vi "GUI_HTT_CTRLv2.vi"() -> ()   [LabVIEW 2013]
uses:
  Shared/GUI_Template/GUI_master/tcp_new_data_event.ctl
  Shared/GUI_Template/GUI_master/tcp new data cluster.ctl
  GUI_TestStand/Fire button.ctl
  <vilib>/Platform/browser.llb/Open URL in Default Browser (string).vi
panel:
  in  "Position.Axis 3::4":dbl caption="Turning M" min=0.0 max=26.0
  in  "Position.Axis 2::4":dbl caption="Delay" min=-20.0 max=48.0
  in  "FilterWheelB1":bool caption="PicoB GUI"
  in  "Search Log":bool caption="PicoL GUI"
  in  "Experiment \n(if, shadow, topjet)":bool caption="PicoL GUI"
  in  "Switcher":bool
  in  "RemoteDesktop":bool caption="PicoL GUI"
  in  "ai_mean.channel 1::13":dbl caption="GenTec" min=0.0 max=0.0 format="%#_6e"
  in  "ai_mean.channel 0::13":dbl caption="Pelliclemeter" min=0.0 max=0.0 format="%#_6e"
  in  "GUIdevice 13":string="HTT_DG645"
  in  "Experiment \n(e-profile, xrays)":bool caption="PicoL GUI"
  in  "IR TC Pointing (17s)":bool caption="PicoL GUI"
  in  "Scatter Depletion":bool caption="PicoL GUI"
  in  "Scatter IR Amps":bool caption="PicoL GUI"
  in  "Drive TC Pt":bool caption="PicoL GUI"
  in  "Gaia Profiles":bool caption="PicoL GUI"
  in  "Gaia Pointing":bool caption="PicoL GUI"
  in  "IR Exp and Comp":bool caption="PicoL GUI"
  in  "HTT Interactive":bool caption="PicoL GUI"
  in  "GUIdevice 12":string="HTT_DG645"
  in  "Delay.Ch C::12":dbl caption="Delay" min=-0.1 max=2.0 format="%#_6e"
  in  "Delay.Ch D::12":dbl caption="Width" min=-0.1 max=2.0 format="%#_6e"
  in  "Amplitude.Ch CD::12":dbl caption="DG645" min=0.5 max=5.0
  in  "Field::1":dbl caption="B-Field" min=0.0 max=10000.0
  in  "Delay.Ch 1::8":dbl caption="Delay" min=0.0 max=10.0 format="%#_6e"
  in  "Width.Ch 1::8":dbl caption="Width" min=0.0 max=1.0 format="%#_6e"
  in  "Amplitude.Ch 1::8":dbl caption="Cam Trig Amp" min=0.0 max=12.0
  in  "Position.Axis 2::6":dbl caption="Prepulse delay" min=-6000.0 max=6000.0
  in  "1Wire GUI":bool caption="PicoL GUI"
  in  "Opt. Spectrometer":bool caption="PicoL GUI"
  in  "SingleCamGUI":bool caption="PicoL GUI"
  in  "Exp Editor":bool caption="PicoL GUI"
  in  "DB Editor":bool caption="PicoL GUI"
  in  "AddColumns":bool caption="PicoL GUI"
  in  "GEECSplot":bool caption="PicoL GUI"
  in  "LVStarter":bool caption="PicoL GUI"
  in  "MasterControl":bool caption="PicoL GUI"
  in  "MagSpecGUI":bool caption="PicoL GUI"
  in  "DailyLog":bool caption="PicoL GUI"
  in  "EnTempLogger":bool caption="PicoL GUI"
  in  "Depletion Cams":bool caption="PicoL GUI"
  in  "D-L-Cams":bool caption="PicoL GUI"
  in  "Position.Axis 2::5":dbl caption="Mode Out z" min=-150.0 max=150.0
  in  "Position.Axis 1::4":dbl caption="Blade" min=-20.0 max=20.0
  out "Temperature::11":dbl caption="Temp Amps" min=0.0 max=500.0 format="%#_3f"
  out "Temperature::10":dbl caption="Temp Gaia" min=0.0 max=500.0 format="%#_3f"
  out "Energy.Channel 0::7":dbl caption="IR Splitmeter" min=0.0 max=20.0 format="%#_3e"
  in  "Amplitude.Ch 5::8":dbl caption="Trigger Amplitude" min=0.0 max=12.0
  in  "Position.Axis 3::5":dbl caption="Mode In z" min=-200.0 max=200.0
  in  "Position.Axis 1::5":dbl caption="Mode Out Wedge" min=-150.0 max=150.0
  out "Position.Axis3::2":dbl caption="Rotation G1" min=-180.0 max=180.0 format="%#_13g"
  out "Position.Axis2::2":dbl caption="Rotation G2" min=-180.0 max=180.0 format="%#_13g"
  in  "Position.Axis1::2":dbl caption="Translation" min=-60000.0 max=60000.0 format="%#_13g"
  in  "PicoL":bool caption="PicoL GUI"
  in  "PicoB":bool caption="PicoB GUI"
  in  "AnalogOutput.Channel 0::9":dbl caption="Pressure Ctrl (V)" min=0.0 max=10.0
  in  "Width.Ch 5::8":dbl caption="Opening time (s)" min=0.0 max=0.025 format="%#_6e"
  in  "Jet enable":bool caption="Jet Enable"
  in  "Jet trigger":bool caption="Jet Trigger"
  in  "Position.Axis 3::3":dbl caption="Jet Z" min=-25.0 max=25.0
  in  "Position.Axis 2::3":dbl caption="Jet Y" min=-25.0 max=25.0
  in  "Position.Axis 1::3":dbl caption="Jet X" min=-25.0 max=25.0
  in  "Position.Axis 3::6":dbl caption="Probe delay" min=-76.0 max=76.0
  in  "GUIdevice 11":string="HTT-Temp-Amps"
  in  "GUIdevice 8":string="HTT-BNC"
  in  "GUIdevice 6":string="HTT-ESP04"
  in  "GUIdevice 5":string="HTT-ESP03"
  in  "Fire Button":T1=TRUE
  out "error IO 2":errorcluster
  out "fire::10":string
  out "tcp data event":T2
  in  "UDP error message":string
  in  "GUIdevice 7":string="HTT-Pulsar"
  in  "GUIdevice 2":string="Aerotech-HTT"
  in  "GUIdevice 10":string="HTT-Temp-Gaia"
  in  "GUIdevice 4":string="HTT-ESP02"
  in  "GUIdevice 1":string="HTT-MagTeslameter-DTM141"
  in  "GUIdevice 3":string="HTT-ESP01"
  in  "GUIdevice 9":string="HTT-HighPressureDAQ"
  in  "Delay.Ch 5::8":dbl caption="Jet timing (s)" min=0.0 max=10.0 format="%#_6e"
  in  "stop":bool
  # "Energy"
  # "CAP"
  # "HTT CONTROL CENTER"
  # "Drive"
  # "Gas Jet"
  # "GUI Collection"
  # "Drive Cameras"
  # "Compressor"
  # "Mode Imager"
  # "Scatter Cameras"
  # "Scatter"
  # "Electronics"
  # "BNC"
  # "Experiment GUIs"
  # "MC Links"
  # "Documentation"
  # "Adjustment GUIs"
  # "Energy Measurements"
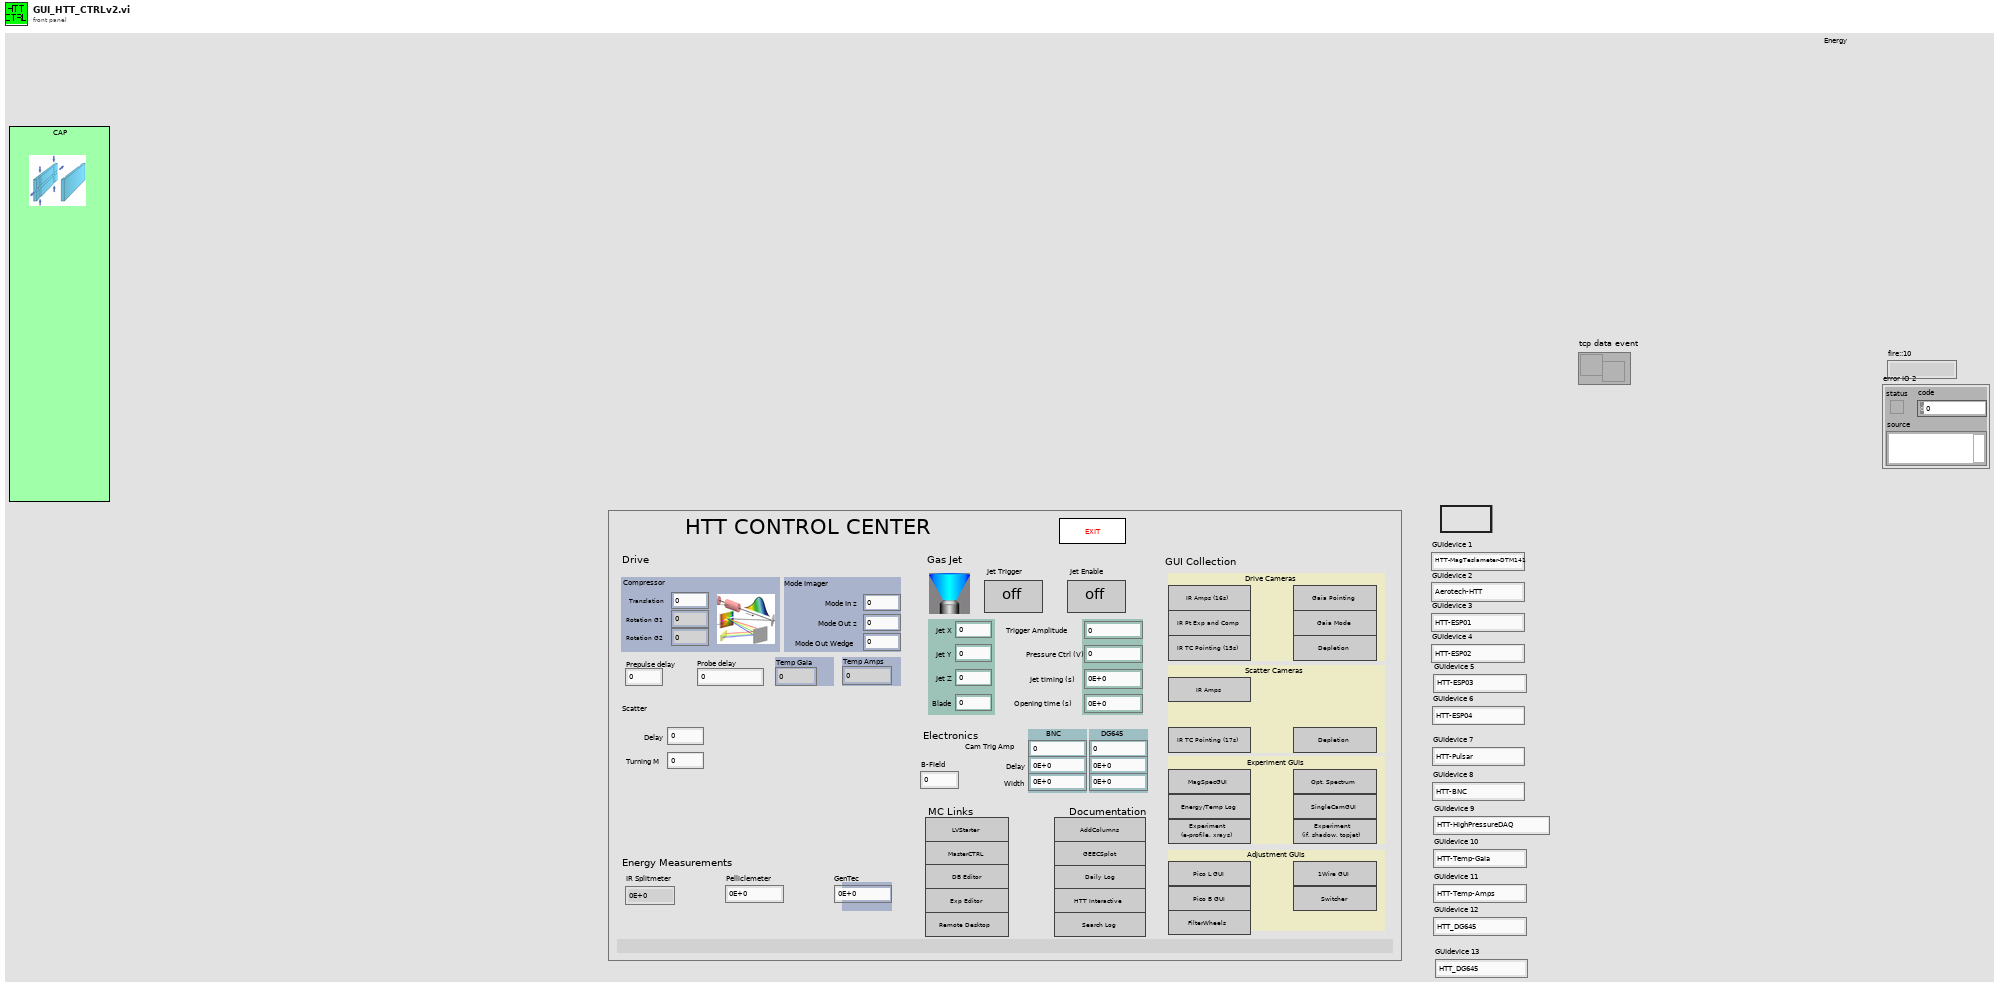
[diagram p1: front panel]
types:
  T1 = typedef "Fire button.ctl" = bool
  T2 = typedef "tcp_new_data_event.ctl" = refnum<user-event>
  T3 = typedef "tcp new data cluster.ctl" = cluster{"EventEnum":enum16{"new data", "connection status update"}, "Device name":string}
  T4 = enum32{"invalid app kind", "Development System", "Run Time System", "Student Edition", "Embedded LabVIEW", "Evaluation", "Custom"}
  T5 = enum32{"Invalid", "Standard", "Closed", "Hidden", "Minimized", "Maximized"}
  T6 = cluster{"Core":cluster{"Current VI Reference":refnum<vi>, "Close Panel on Exit?":bool}, "Heater timing offset":dbl, "Discharge timing offset":dbl, "Jet trigger":bool, "Tik1":u32, "Tik2":u32, "Fire Continues Allowed":bool, "Jet enable":bool}
  T7 = cluster{"Current VI Reference":refnum<vi>, "Close Panel on Exit?":bool}
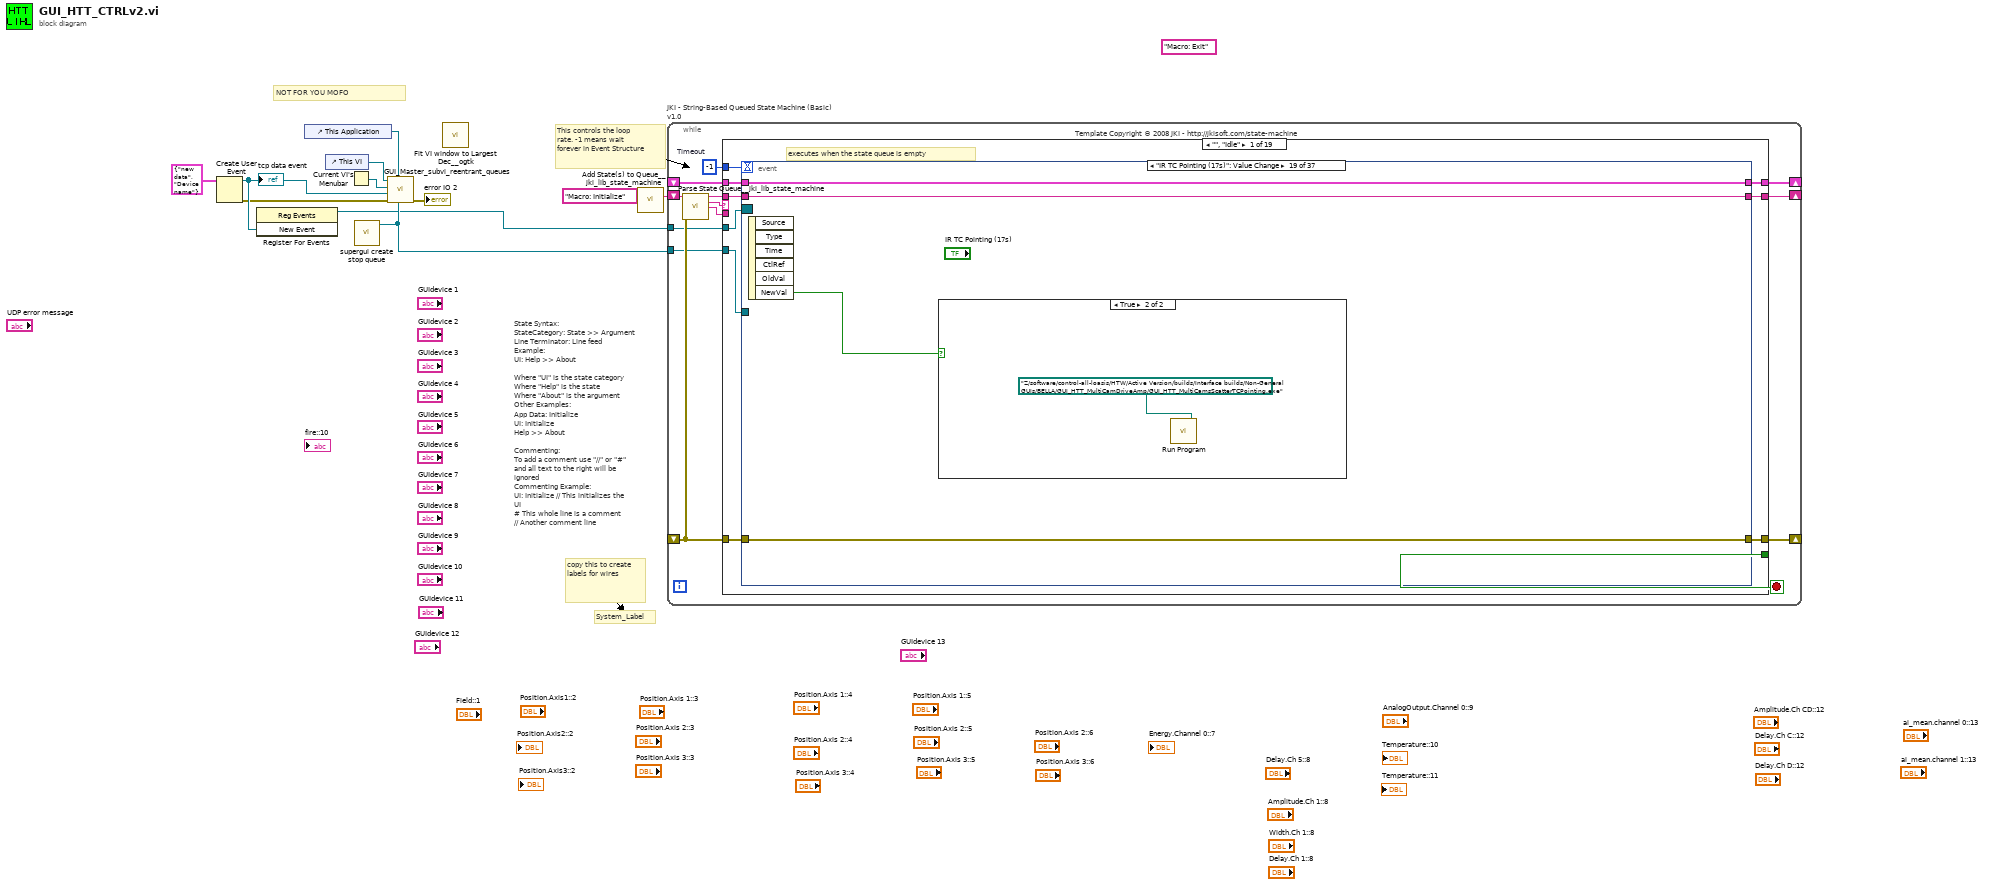
[diagram p0: block diagram]
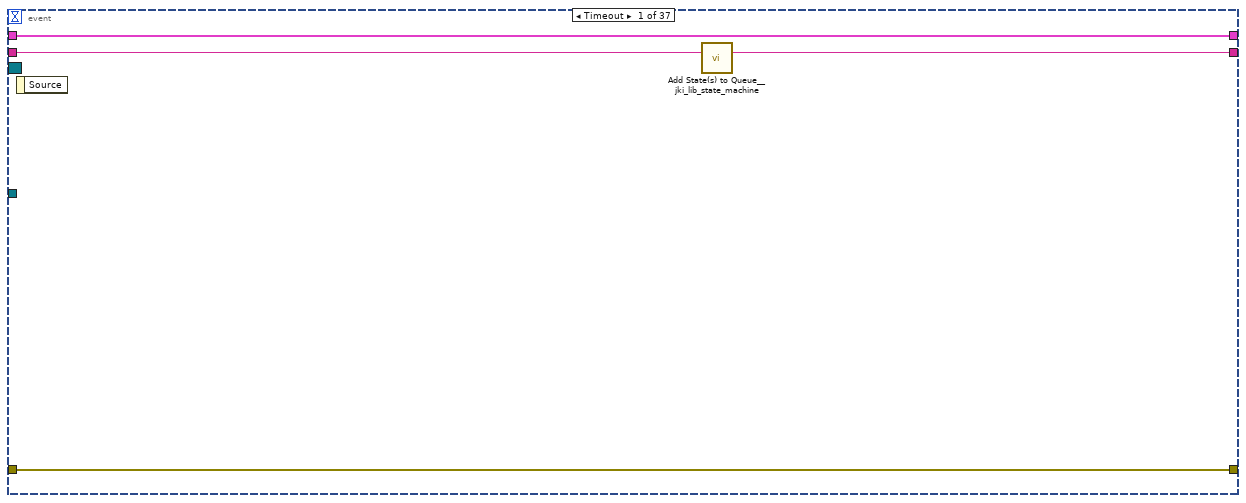
[diagram p2: hidden frame]
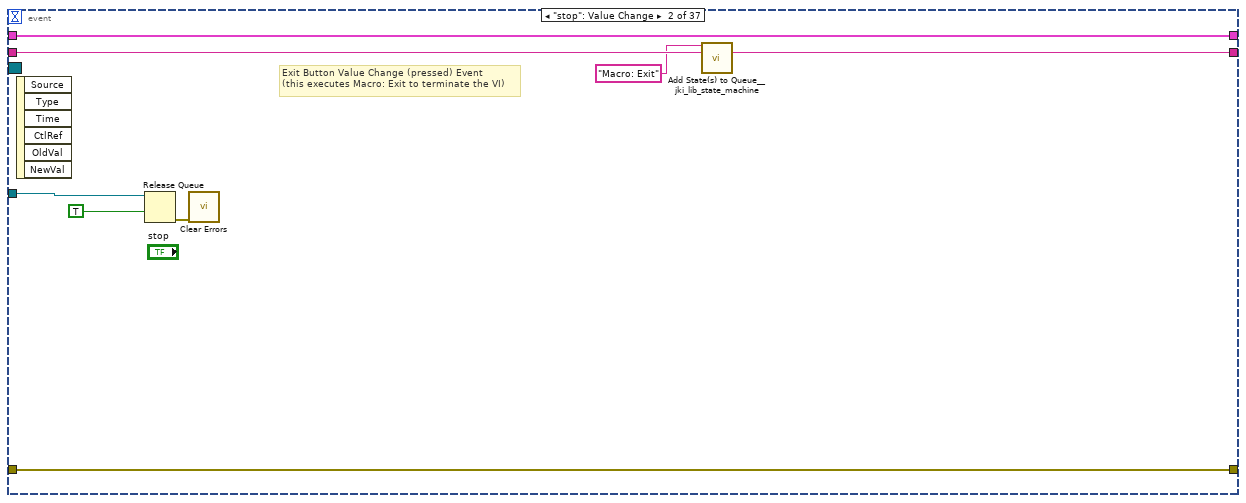
[diagram p3: hidden frame]
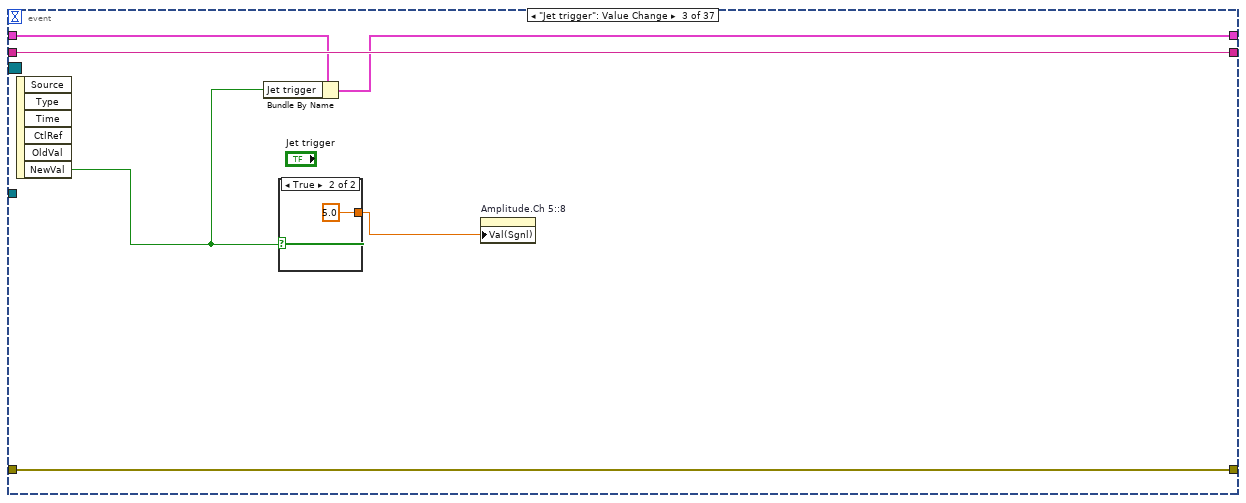
[diagram p4: hidden frame]
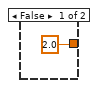
[diagram p5: hidden frame]
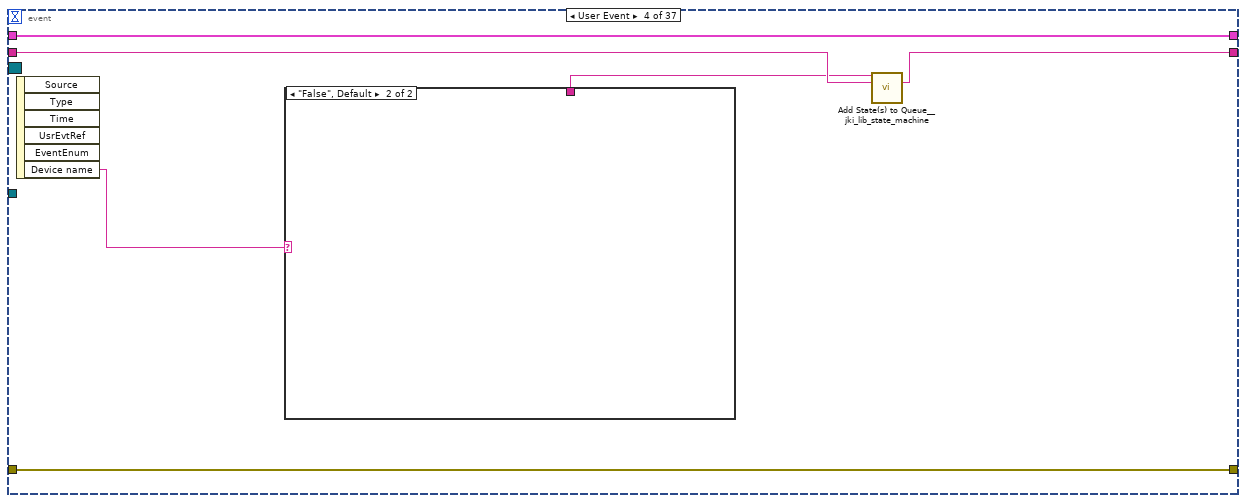
[diagram p6: hidden frame]
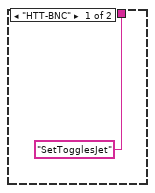
[diagram p7: hidden frame]
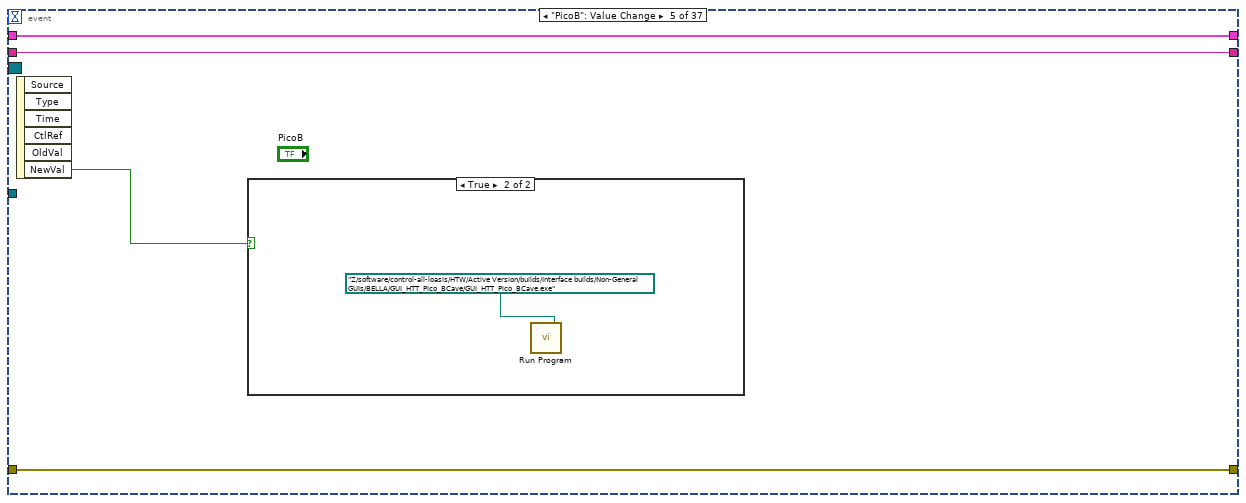
[diagram p8: hidden frame]
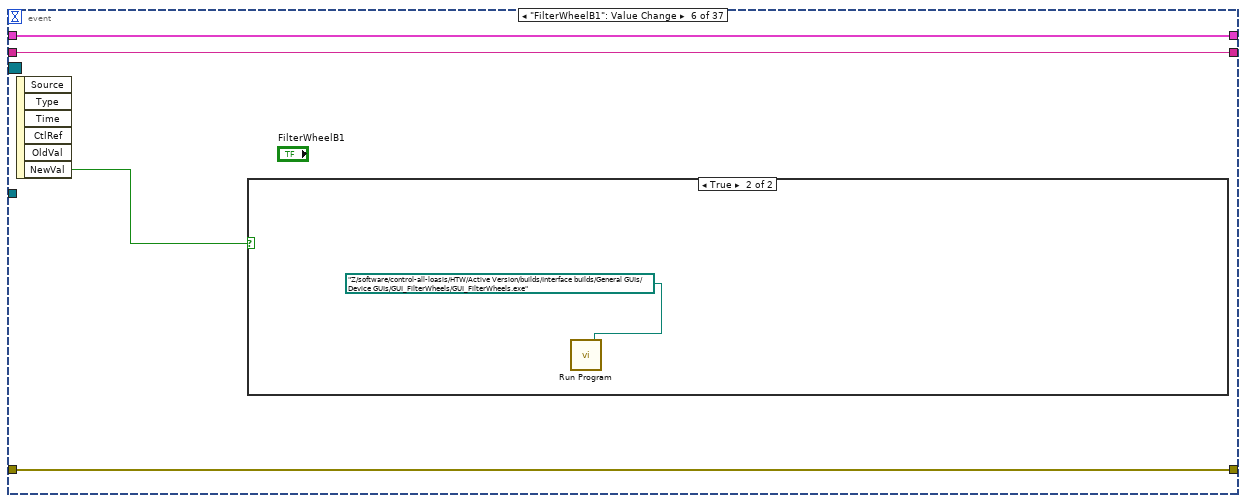
[diagram p10: hidden frame]
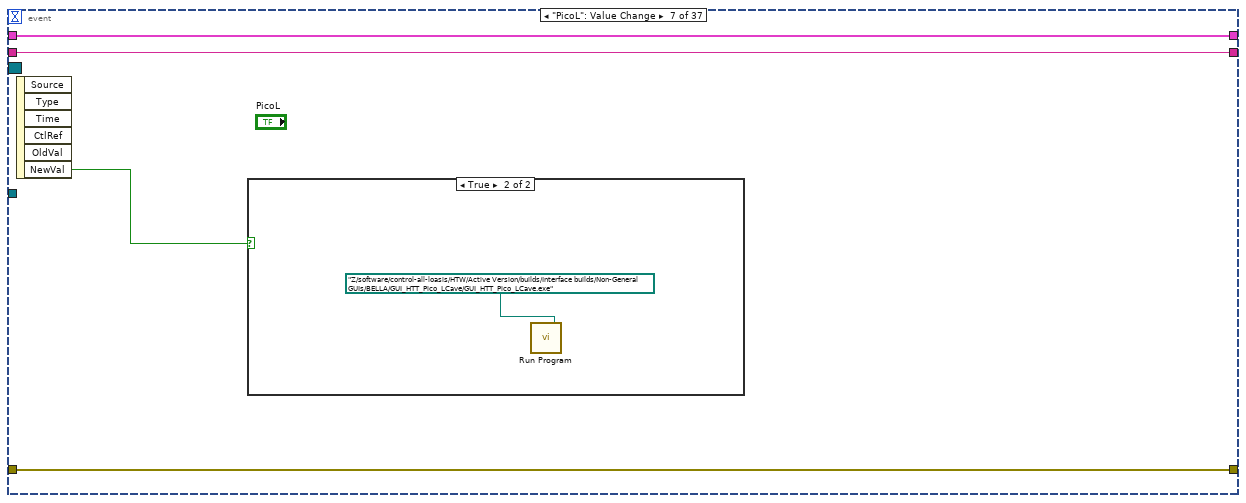
[diagram p12: hidden frame]
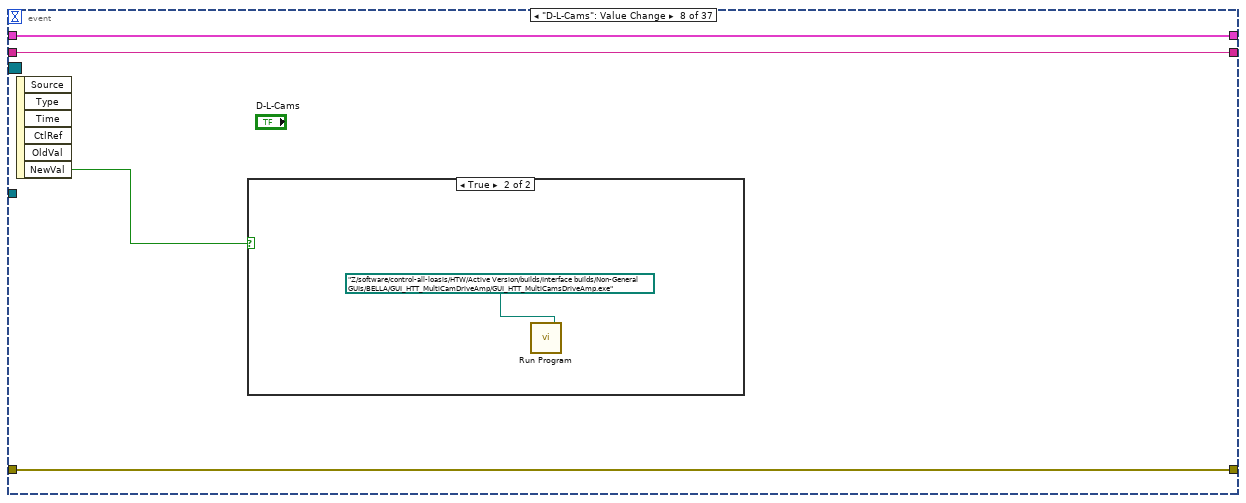
[diagram p14: hidden frame]
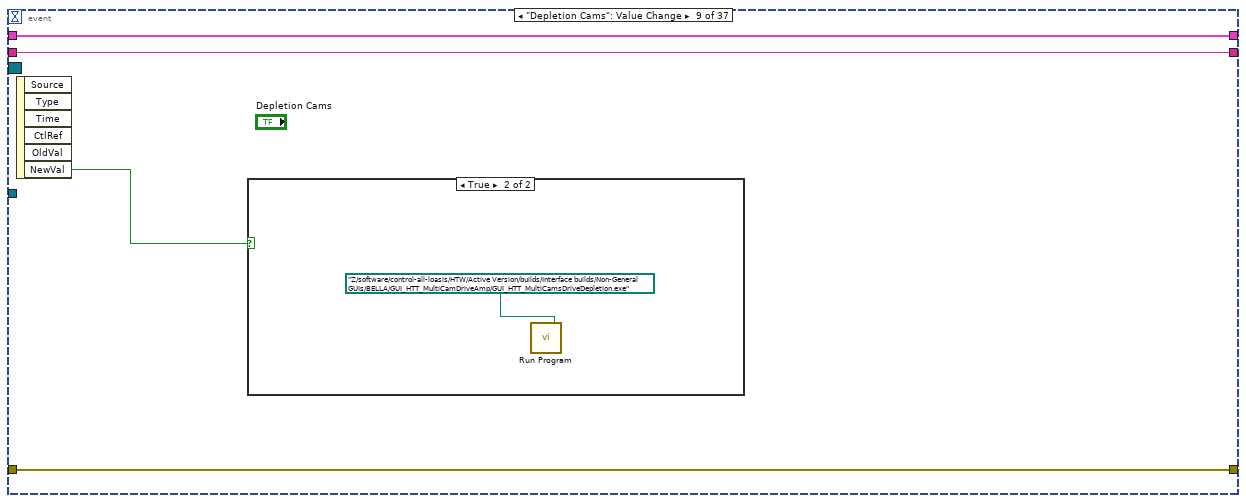
[diagram p16: hidden frame]
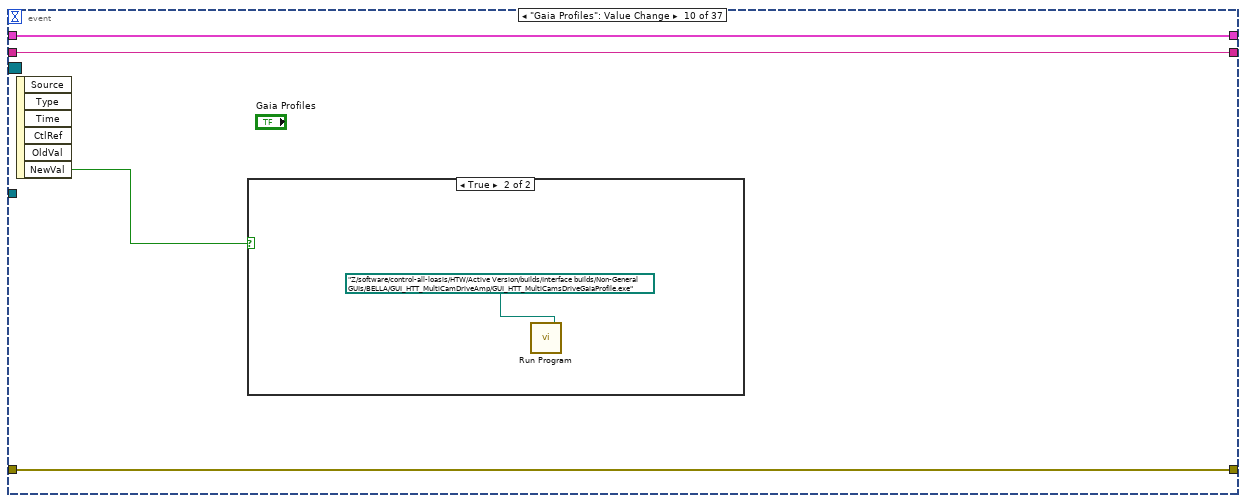
[diagram p18: hidden frame]
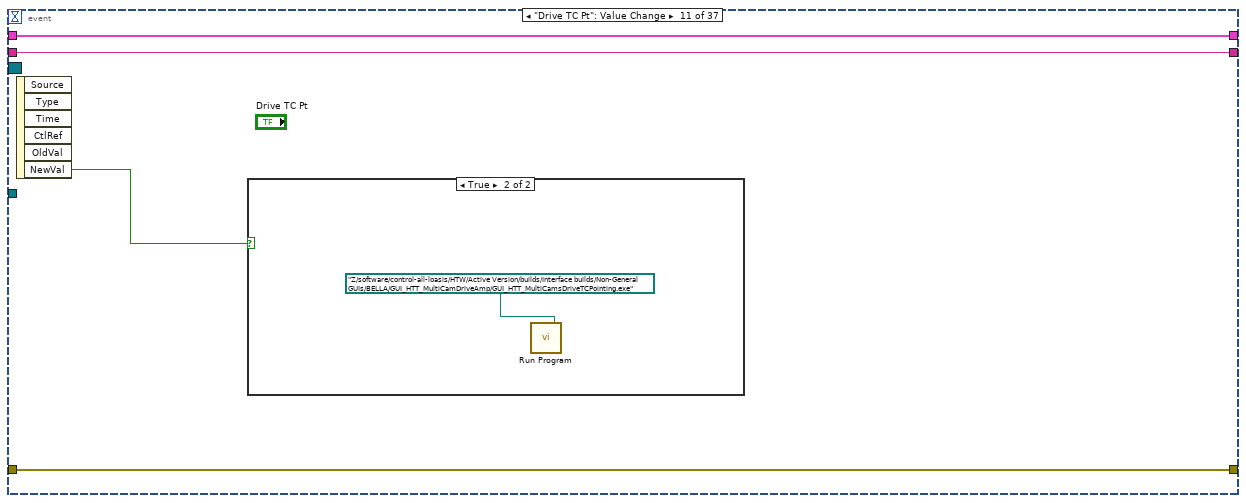
[diagram p20: hidden frame]
diagram:
  (unwired) "Macro: Exit"
  # "State Syntax:\nStateCategory: State >> Argument\nLine Terminator: Line feed\nExample:\nUI: Help >> About\n\nWhere \"UI\" is the state category\nWhere \"Help\" is the state\nWhere \"About\" is the argument\nOther Examples:\nApp Data: Initialize\nUI: Initialize\nHelp >> About\n\nCommenting:\nTo add a comment use \"//\" or \"#\" and all text to the right will be ignored\nCommenting Example:\nUI: Initialize // This initializes the UI\n# This whole line is a comment\n// Another comment line"
  # "copy this to create labels for wires"
  # "This controls the loop rate. -1 means wait forever in Event Structure"
  # "System_Label"
  # "NOT FOR YOU MOFO"
  n1 = Create User Event(user event datatype=T3 {"EventEnum"=enum."new data", "Device name"="Device name"} ("New Event")) -> (user event=w10:refnum<user-event>, error out=w9:errorcluster)  [unwired: 1 in]
  "tcp data event" <- w10
  n2 = register-events(w10) -> (reference out=w1:refnum<event-registration>)  [unwired: 2 in, 1 out]
  n3 = control-ref of="This Application"() -> (w11:refnum<vi>)
  n4 = control-ref of="This VI"() -> (w5:refnum<vi>)
  n5 = Current VI's Menubar() -> (w7:refnum<k9>)
  n6 = call "supergui create stop queue.vi"() -> ("STOP Queue out"=w2:refnum<queue>)  [unwired: 11 in]
  n7 = call "GUI_Master_subvi_reentrant_queues.vi"("STOP Queue in"=w2, "This Application"=w11, "error in (no error)"=w9, "tcp data event"=w10, "Caller menu reference"=w7, "Caller VI ref"=w5) -> ("error out"=→"error IO 2":errorcluster)  [unwired: 5 in]
  n8 = call <userlib>:"Fit VI window to Largest Dec__ogtk.vi"() -> ()  [unwired: 6 in, 2 out]
  n9 = call <vilib>:"Add State(s) to Queue__jki_lib_state_machine.vi"("State(s) in (\"\")"="Macro: Initialize") -> ("States Out"=w3:string)  [unwired: 14 in]
  n10 = while "JKI - String-Based Queued State Machine (Basic) v1.0" {
    shift-right: [w17] -> _
    shift-left: _ -> [w16]
    shift-right: [w20] -> _
    shift-left: _ -> [w14]
    shift-right: [w19] -> _
    shift-left: w3 -> [w21]
    tunnel: w1 -> [w13]
    tunnel: w2 -> [w12]
    stop <- w18 stop-if-true
    w15 = -1  # Timeout
    # "Template Copyright © 2008 JKI - http://jkisoft.com/state-machine"
    n11 = call <vilib>:"Parse State Queue__jki_lib_state_machine.vi"("State Queue"=w21, "Error In (no error)"=w14) -> ("Remaining States"=w23:string, "Current State"=w24:string, "Arguments"=w22:string)  [unwired: 11 in]
    n12 = case shown="\"\", \"Idle\"" w24 {
      selector: w24 -> [_ _ _ w249 _ _ _ _ _ _ _ _ _ _ _ _ _ _ _]
      tunnel: w23 -> [w33 w243 w248 w253 w271 w277 w282 w286 w298 w304 w308 w312 w318 w329 w355 w360 w370 w374 w380]
      tunnel: w22 -> [_ _ _ _ _ _ _ _ _ _ _ _ w313 w323 _ _ _ _ _]
      tunnel: w16 -> [w31 w244 w245 w251 w262 w274 w280 w283 _ w299 w305 w310 w316 w325 w352 w357 w367 w371 w378]
      tunnel: [w30 w242 w246 w255 w268 errorcluster {"status"=FALSE, "code"=0, "source"=""} ("error out") w279 w284 w295 w300 w306 w309 w314 w326 w353 w358 w368 w372 w375] -> w20
      tunnel: w14 -> [w29 w242 w246 w254 w268 w273 w279 w284 w295 w301 w306 w309 w315 w327 w353 w358 w368 w372 w376]
      tunnel: [w32 w243 w247 w252 w270 w276 w281 w285 w297 w303 w307 w311 w317 w328 w354 w359 w369 w373 w379] -> w19
      tunnel: [_ _ _ _ _ _ TRUE _ _ _ _ _ _ _ _ _ _ _ _] -> w18
      tunnel: [w25 w244 w245 w251 w269 w274 w280 w283 w296 w299 w305 w310 w316 w325 w352 w357 w367 w371 w378] -> w17
      tunnel: w15 -> [w28 _ _ _ _ _ _ _ _ _ _ _ _ _ _ _ _ _ _]
      tunnel: w13 -> [w27 _ _ _ _ _ _ _ _ _ _ _ _ _ _ _ _ _ _]
      tunnel: w12 -> [w26 _ _ _ _ _ _ _ _ _ _ _ _ _ _ _ _ _ _]
      frame "", "Idle" {
        # "executes when the state queue is empty"
        n13 = event shown="[18] \"IR TC Pointing (17s)\": Value Change" {
          selector: w27 -> [_ _ _ _ _ _ _ _ _ _ _ _ _ _ _ _ _ _ _ _ _ _ _ _ _ _ _ _ _ _ _ _ _ _ _ _ _]
          dyn-events: _ -> [_ _ _ _ _ _ _ _ _ _ _ _ _ _ _ _ _ _ _ _ _ _ _ _ _ _ _ _ _ _ _ _ _ _ _ _ _]
          timeout: w28 -> [_ _ _ _ _ _ _ _ _ _ _ _ _ _ _ _ _ _ _ _ _ _ _ _ _ _ _ _ _ _ _ _ _ _ _ _ _]
          tunnel: w33 -> [w37 w45 w51 w57 w64 w69 w74 w79 w84 w89 w94 w99 w104 w109 w114 w119 w124 w129 w134 w139 w144 w149 w154 w159 w164 w169 w174 w179 w184 w189 w194 w199 w204 w209 w216 w220 w229]
          tunnel: [w36 w44 w51 w56 w64 w69 w74 w79 w84 w89 w94 w99 w104 w109 w114 w119 w124 w129 w134 w139 w144 w149 w154 w159 w164 w169 w174 w179 w184 w189 w194 w199 w204 w209 w216 w221 w228] -> w32
          tunnel: w31 -> [w34 w42 w50 w58 w61 w66 w71 w76 w81 w86 w91 w96 w101 w106 w111 w116 w121 w126 w131 w136 w141 w146 w151 w156 w161 w166 w171 w176 w181 w186 w191 w196 w201 w206 w215 w223 w226]
          tunnel: [w35 w43 w47 w55 w62 w67 w72 w77 w82 w87 w92 w97 w102 w107 w112 w117 w122 w127 w132 w137 w142 w147 w152 w157 w162 w167 w172 w177 w182 w187 w192 w197 w202 w207 w211 w222 w227] -> w30
          tunnel: w29 -> [w35 w43 w47 w55 w62 w67 w72 w77 w82 w87 w92 w97 w102 w107 w112 w117 w122 w127 w132 w137 w142 w147 w152 w157 w162 w167 w172 w177 w182 w187 w192 w197 w202 w207 w211 w222 w227]
          tunnel: [w34 w42 w49 w58 w61 w66 w71 w76 w81 w86 w91 w96 w101 w106 w111 w116 w121 w126 w131 w136 w141 w146 w151 w156 w161 w166 w171 w176 w181 w186 w191 w196 w201 w206 w214 w223 w226] -> w25
          tunnel: w26 -> [_ w39 _ _ _ _ _ _ _ _ _ _ _ _ _ _ _ _ _ _ _ _ _ _ _ _ _ _ _ _ _ _ _ _ _ _ _]
          event Timeout {
            n14 = event-data() -> ()  [unwired: 1 in, 1 out]
            n15 = call <vilib>:"Add State(s) to Queue__jki_lib_state_machine.vi"("State(s) in (\"\")"=w37) -> ("States Out"=w36:string)  [unwired: 14 in]
          }
          event "stop": Value Change {
            # "Exit Button Value Change (pressed) Event\n(this executes Macro: Exit to terminate the VI)"
            n16 = event-data() -> ()  [unwired: 1 in, 6 out]
            n17 = Release Queue(queue=w39, force destroy? (F)=TRUE) -> (error out=w40:errorcluster)  [unwired: 1 in, 2 out]
            n18 = call <vilib>:"Clear Errors.vi"("error in (no error)"=w40) -> ()  [unwired: 6 in, 1 out]
            n19 = call <vilib>:"Add State(s) to Queue__jki_lib_state_machine.vi"("State(s) in Front (\"\")"="Macro: Exit", "State(s) in (\"\")"=w45) -> ("States Out"=w44:string)  [unwired: 13 in]
          }
          event "Jet trigger": Value Change {
            n20 = event-data() -> ("NewVal"=w48:bool)  [unwired: 1 in, 5 out]
            n21 = Bundle By Name(cluster=w50, "Jet trigger"=w48) -> (w49:T6)
            n22 = case shown="True" w48 {
              tunnel: [2.0 ("Amplitude.Ch CD::10") 5.0 ("Amplitude.Ch CD::10")] -> w46
              frame False {
              }
              frame True {
              }
            }
            n23 = property on="Amplitude.Ch 5::8" class="DigNum (strict)"("Val(Sgnl)"=w46) -> ()  [unwired: 2 in, 2 out]
          }
          event User Event {
            n24 = event-data() -> ("Device name"=w59:string)  [unwired: 1 in, 5 out]
            n25 = case shown="\"False\", Default" w59 {
              tunnel: ["SetTogglesJet" _] -> w54
              frame "HTT-BNC" {
              }
              frame "False", Default {
              }
            }
            n26 = call <vilib>:"Add State(s) to Queue__jki_lib_state_machine.vi"("State(s) in Front (\"\")"=w54, "State(s) in (\"\")"=w57) -> ("States Out"=w56:string)  [unwired: 13 in]
          }
          event "PicoB": Value Change {
            n27 = event-data() -> ("NewVal"=w63:bool)  [unwired: 1 in, 5 out]
            n28 = case shown="True" w63 {
              frame False {
              }
              frame True {
                n29 = call "Run Program.vi"("Program Path"=path "Z:/software/control-all-loasis/HTW/Active Version/builds/Interface builds/Non-General GUIs/BELLA/GUI_HTT_Pico_BCave/GUI_HTT_Pico_BCave.exe") -> ()  [unwired: 1 in]
              }
            }
          }
          event "FilterWheelB1": Value Change {
            n30 = event-data() -> ("NewVal"=w68:bool)  [unwired: 1 in, 5 out]
            n31 = case shown="True" w68 {
              frame False {
              }
              frame True {
                n32 = call "Run Program.vi"("Program Path"=path "Z:/software/control-all-loasis/HTW/Active Version/builds/Interface builds/General GUIs/Device GUIs/GUI_FilterWheels/GUI_FilterWheels.exe") -> ()  [unwired: 1 in]
              }
            }
          }
          event "PicoL": Value Change {
            n33 = event-data() -> ("NewVal"=w73:bool)  [unwired: 1 in, 5 out]
            n34 = case shown="True" w73 {
              frame False {
              }
              frame True {
                n35 = call "Run Program.vi"("Program Path"=path "Z:/software/control-all-loasis/HTW/Active Version/builds/Interface builds/Non-General GUIs/BELLA/GUI_HTT_Pico_LCave/GUI_HTT_Pico_LCave.exe") -> ()  [unwired: 1 in]
              }
            }
          }
          event "D-L-Cams": Value Change {
            n36 = event-data() -> ("NewVal"=w78:bool)  [unwired: 1 in, 5 out]
            n37 = case shown="True" w78 {
              frame False {
              }
              frame True {
                n38 = call "Run Program.vi"("Program Path"=path "Z:/software/control-all-loasis/HTW/Active Version/builds/Interface builds/Non-General GUIs/BELLA/GUI_HTT_MultiCamDriveAmp/GUI_HTT_MultiCamsDriveAmp.exe") -> ()  [unwired: 1 in]
              }
            }
          }
          event "Depletion Cams": Value Change {
            n39 = event-data() -> ("NewVal"=w83:bool)  [unwired: 1 in, 5 out]
            n40 = case shown="True" w83 {
              frame False {
              }
              frame True {
                n41 = call "Run Program.vi"("Program Path"=path "Z:/software/control-all-loasis/HTW/Active Version/builds/Interface builds/Non-General GUIs/BELLA/GUI_HTT_MultiCamDriveAmp/GUI_HTT_MultiCamsDriveDepletion.exe") -> ()  [unwired: 1 in]
              }
            }
          }
          event "Gaia Profiles": Value Change {
            n42 = event-data() -> ("NewVal"=w88:bool)  [unwired: 1 in, 5 out]
            n43 = case shown="True" w88 {
              frame False {
              }
              frame True {
                n44 = call "Run Program.vi"("Program Path"=path "Z:/software/control-all-loasis/HTW/Active Version/builds/Interface builds/Non-General GUIs/BELLA/GUI_HTT_MultiCamDriveAmp/GUI_HTT_MultiCamsDriveGaiaProfile.exe") -> ()  [unwired: 1 in]
              }
            }
          }
          event "Drive TC Pt": Value Change {
            n45 = event-data() -> ("NewVal"=w93:bool)  [unwired: 1 in, 5 out]
            n46 = case shown="True" w93 {
              frame False {
              }
              frame True {
                n47 = call "Run Program.vi"("Program Path"=path "Z:/software/control-all-loasis/HTW/Active Version/builds/Interface builds/Non-General GUIs/BELLA/GUI_HTT_MultiCamDriveAmp/GUI_HTT_MultiCamsDriveTCPointing.exe") -> ()  [unwired: 1 in]
              }
            }
          }
          event "Scatter IR Amps": Value Change {
            n48 = event-data() -> ("NewVal"=w98:bool)  [unwired: 1 in, 5 out]
            n49 = case shown="True" w98 {
              frame False {
              }
              frame True {
                n50 = call "Run Program.vi"("Program Path"=path "Z:/software/control-all-loasis/HTW/Active Version/builds/Interface builds/Non-General GUIs/BELLA/GUI_HTT_MultiCamScatterAmp/GUI_HTT_MultiCamsScatterAmp.exe") -> ()  [unwired: 1 in]
              }
            }
          }
          event "Scatter Depletion": Value Change {
            n51 = event-data() -> ("NewVal"=w103:bool)  [unwired: 1 in, 5 out]
            n52 = case shown="True" w103 {
              frame False {
              }
              frame True {
                n53 = call "Run Program.vi"("Program Path"=path "Z:/software/control-all-loasis/HTW/Active Version/builds/Interface builds/Non-General GUIs/BELLA/GUI_HTT_MultiCamScatterAmp/GUI_HTT_MultiCamsScatterAmp.exe") -> ()  [unwired: 1 in]
              }
            }
          }
          event "IR Exp and Comp": Value Change {
            n54 = event-data() -> ("NewVal"=w108:bool)  [unwired: 1 in, 5 out]
            n55 = case shown="True" w108 {
              frame False {
              }
              frame True {
                n56 = call "Run Program.vi"("Program Path"=path "Z:/software/control-all-loasis/HTW/Active Version/builds/Interface builds/Non-General GUIs/BELLA/GUI_HTT_MultiCamDriveAmp/GUI_HTT_MultiCamsDriveExpAndComp.exe") -> ()  [unwired: 1 in]
              }
            }
          }
          event "Gaia Pointing": Value Change {
            n57 = event-data() -> ("NewVal"=w113:bool)  [unwired: 1 in, 5 out]
            n58 = case shown="True" w113 {
              frame False {
              }
              frame True {
                n59 = call "Run Program.vi"("Program Path"=path "Z:/software/control-all-loasis/HTW/Active Version/builds/Interface builds/Non-General GUIs/BELLA/GUI_HTT_MultiCamDriveGaiaPointing/GUI_HTT_MultiCamsDriveGaiaPointing.exe") -> ()  [unwired: 1 in]
              }
            }
          }
          event "EnTempLogger": Value Change {
            n60 = event-data() -> ("NewVal"=w118:bool)  [unwired: 1 in, 5 out]
            n61 = case shown="True" w118 {
              frame False {
              }
              frame True {
                n62 = call "Run Program.vi"("Program Path"=path "Z:/software/control-all-loasis/HTW/Active Version/builds/Interface builds/Non-General GUIs/BELLA/GUI_HTT_Logger/GUI_HTT_Logger.exe") -> ()  [unwired: 1 in]
              }
            }
          }
          event "1Wire GUI": Value Change {
            n63 = event-data() -> ("NewVal"=w123:bool)  [unwired: 1 in, 5 out]
            n64 = case shown="True" w123 {
              frame False {
              }
              frame True {
                n65 = call "Run Program.vi"("Program Path"=path "Z:/software/control-all-loasis/HTW/Active Version/builds/Interface builds/Non-General GUIs/BELLA/GUI_HTT_1Wire/GUI_HTT_1Wire.exe") -> ()  [unwired: 1 in]
              }
            }
          }
          event "MagSpecGUI": Value Change {
            n66 = event-data() -> ("NewVal"=w128:bool)  [unwired: 1 in, 5 out]
            n67 = case shown="True" w128 {
              frame False {
              }
              frame True {
                n68 = call "Run Program.vi"("Program Path"=path "Z:/software/control-all-loasis/HTW/Active Version/builds/Interface builds/Non-General GUIs/BELLA/GUI_HTT_MultiCamDriveAmp/GUI_HTT_MultiCamsDriveMagSpec.exe") -> ()  [unwired: 1 in]
              }
            }
          }
          event "IR TC Pointing (17s)": Value Change {
            n69 = event-data() -> ("NewVal"=w133:bool)  [unwired: 1 in, 5 out]
            n70 = case shown="True" w133 {
              frame False {
              }
              frame True {
                n71 = call "Run Program.vi"("Program Path"=path "Z:/software/control-all-loasis/HTW/Active Version/builds/Interface builds/Non-General GUIs/BELLA/GUI_HTT_MultiCamDriveAmp/GUI_HTT_MultiCamsScatterTCPointing.exe") -> ()  [unwired: 1 in]
              }
            }
          }
          event "Experiment \n(e-profile, xrays)": Value Change {
            n72 = event-data() -> ("NewVal"=w138:bool)  [unwired: 1 in, 5 out]
            n73 = case shown="True" w138 {
              frame False {
              }
              frame True {
                n74 = call "Run Program.vi"("Program Path"=path "Z:/software/control-all-loasis/HTW/Active Version/builds/Interface builds/Non-General GUIs/BELLA/GUI_HTT_MultiCamDriveAmp/GUI_HTT_MultiCamsDriveExperiment1.exe") -> ()  [unwired: 1 in]
              }
            }
          }
          event "Experiment \n(if, shadow, topjet)": Value Change {
            n75 = event-data() -> ("NewVal"=w143:bool)  [unwired: 1 in, 5 out]
            n76 = case shown="True" w143 {
              frame False {
              }
              frame True {
                n77 = call "Run Program.vi"("Program Path"=path "Z:/software/control-all-loasis/HTW/Active Version/builds/Interface builds/Non-General GUIs/BELLA/GUI_HTT_MultiCamDriveAmp/GUI_HTT_MultiCamsDriveExperiment2.exe") -> ()  [unwired: 1 in]
              }
            }
          }
          event "MasterControl": Value Change {
            n78 = event-data() -> ("NewVal"=w148:bool)  [unwired: 1 in, 5 out]
            n79 = case shown="True" w148 {
              frame False {
              }
              frame True {
                n80 = call "Run Program.vi"("Program Path"=path "Z:/software/control-all-loasis/HTW/Active Version/builds/Interface builds/General GUIs/MC/Master Control/Master Control.exe") -> ()  [unwired: 1 in]
              }
            }
          }
          event "LVStarter": Value Change {
            n81 = event-data() -> ("NewVal"=w153:bool)  [unwired: 1 in, 5 out]
            n82 = case shown="True" w153 {
              frame False {
              }
              frame True {
                n83 = call "Run Program.vi"("Program Path"=path "Z:/software/control-all-loasis/HTW/Active Version/builds/Interface builds/General GUIs/MC/LVstarter/LVstarter.exe") -> ()  [unwired: 1 in]
              }
            }
          }
          event "Switcher": Value Change {
            n84 = event-data() -> ("NewVal"=w158:bool)  [unwired: 1 in, 5 out]
            n85 = case shown="True" w158 {
              frame False {
              }
              frame True {
                n86 = call "Run Program.vi"("Program Path"=path "Z:/software/control-all-loasis/HTW/Active Version/builds/Interface builds/Non-General GUIs/BELLA/GUI_HTT_Switcher/GUI_HTT_Switcher.exe") -> ()  [unwired: 1 in]
              }
            }
          }
          event "GEECSplot": Value Change {
            n87 = event-data() -> ("NewVal"=w163:bool)  [unwired: 1 in, 5 out]
            n88 = case shown="True" w163 {
              frame False {
              }
              frame True {
                n89 = call "Run Program.vi"("Program Path"=path "Z:/software/HTT/GEECSplotter 20180926/GEECSplotter.exe") -> ()  [unwired: 1 in]
              }
            }
          }
          event "AddColumns": Value Change {
            n90 = event-data() -> ("NewVal"=w168:bool)  [unwired: 1 in, 5 out]
            n91 = case shown="True" w168 {
              frame False {
              }
              frame True {
                n92 = call "Run Program.vi"("Program Path"=path "Z:/software/HTT/Add columns to Masterlog 20180703/Add columns to Masterlog.exe") -> ()  [unwired: 1 in]
              }
            }
          }
          event "DB Editor": Value Change {
            n93 = event-data() -> ("NewVal"=w173:bool)  [unwired: 1 in, 5 out]
            n94 = case shown="True" w173 {
              frame False {
              }
              frame True {
                n95 = call "Run Program.vi"("Program Path"=path "Z:/software/control-all-loasis/HTW/Active Version/builds/Interface builds/General GUIs/Database editor/Database editor.exe") -> ()  [unwired: 1 in]
              }
            }
          }
          event "Exp Editor": Value Change {
            n96 = event-data() -> ("NewVal"=w178:bool)  [unwired: 1 in, 5 out]
            n97 = case shown="True" w178 {
              frame False {
              }
              frame True {
                n98 = call "Run Program.vi"("Program Path"=path "Z:/software/control-all-loasis/HTW/Active Version/builds/Interface builds/General GUIs/Database editor/Expt_Devices_GUI.exe") -> ()  [unwired: 1 in]
              }
            }
          }
          event "SingleCamGUI": Value Change {
            n99 = event-data() -> ("NewVal"=w183:bool)  [unwired: 1 in, 5 out]
            n100 = case shown="True" w183 {
              frame False {
              }
              frame True {
                n101 = call "Run Program.vi"("Program Path"=path "Z:/software/control-all-loasis/HTW/Active Version/builds/Interface builds/General GUIs/Device GUIs/GUI_Cameras/GUI_Cameras.exe") -> ()  [unwired: 1 in]
              }
            }
          }
          event "Opt. Spectrometer": Value Change {
            n102 = event-data() -> ("NewVal"=w188:bool)  [unwired: 1 in, 5 out]
            n103 = case shown="True" w188 {
              frame False {
              }
              frame True {
                n104 = call "Run Program.vi"("Program Path"=path "Z:/software/control-all-loasis/HTW/Active Version/builds/Interface builds/Non-General GUIs/BELLA/GUI_HTT_HamamatsuSpec/GUI_HTT_HamamatsuSpec.exe") -> ()  [unwired: 1 in]
              }
            }
          }
          event "RemoteDesktop": Value Change {
            n105 = event-data() -> ("NewVal"=w193:bool)  [unwired: 1 in, 5 out]
            n106 = case shown="True" w193 {
              frame False {
              }
              frame True {
                n107 = call "Run Program.vi"("Program Path"=path "C:/Windows/System32/mstsc.exe") -> ()  [unwired: 1 in]
              }
            }
          }
          event "DailyLog": Value Change {
            n108 = event-data() -> ("NewVal"=w198:bool)  [unwired: 1 in, 5 out]
            n109 = case shown="True" w198 {
              frame False {
              }
              frame True {
                n110 = call-poly <vilib>:"Open URL in Default Browser.vi"("URL"="https://docs.google.com/document/d/1W41t9HHThLxJNgKAdgHl8eoaQaAGTmxKu770EZ7fHZA/edit#") -> ()  [unwired: 5 in, 2 out]
              }
            }
          }
          event "HTT Interactive": Value Change {
            n111 = event-data() -> ("NewVal"=w203:bool)  [unwired: 1 in, 5 out]
            n112 = case shown="True" w203 {
              frame False {
              }
              frame True {
                n113 = call-poly <vilib>:"Open URL in Default Browser.vi"("URL"="https://docs.google.com/presentation/d/1vde03GLRziloe-kxBmiBfXX4-hwSL2uU9dDMmq9JgxY/edit?usp=sharing") -> ()  [unwired: 5 in, 2 out]
              }
            }
          }
          event "Search Log": Value Change {
            n114 = event-data() -> ("NewVal"=w208:bool)  [unwired: 1 in, 5 out]
            n115 = case shown="True" w208 {
              frame False {
              }
              frame True {
                n116 = call-poly <vilib>:"Open URL in Default Browser.vi"("URL"="https://docs.google.com/spreadsheets/d/1wR7To7WJHrQNP-2Id8ScCGPPim0LYwsaw_KNOLmAjJY/edit?usp=sharing") -> ()  [unwired: 5 in, 2 out]
              }
            }
          }
          event "Jet enable": Value Change {
            # "For instructions on how to use the JKI State Machine, examples and video tutorials, visit:\nhttp://jkisoft.com/state-machine/\n\nJKI State Machine™\nhttp://jkisoft.com/state-machine/\nCopyright (C) 2005-2008, JKI <info@jkisoft.com>\nALL RIGHTS RESERVED"
            n117 = event-data() -> ("NewVal"=w213:bool)  [unwired: 1 in, 5 out]
            n118 = case shown="True" w213 {
              tunnel: [0.0 ("opening Time") 0.002 ("opening Time")] -> w212
              frame False {
              }
              frame True {
              }
            }
            n119 = Bundle By Name(cluster=w215, "Jet enable"=w213) -> (w214:T6)
            n120 = property on="Width.Ch 5::8" class="DigNum (strict)"("Val(Sgnl)"=w212) -> ()  [unwired: 2 in, 2 out]
          }
          event Value Change {
            n121 = event-data() -> ()  [unwired: 1 in, 6 out]
            n122 = call <vilib>:"Add State(s) to Queue__jki_lib_state_machine.vi"("State(s) in Front (\"\")"="Action: Fire" ("State(s) in Front (\"\")"), "State(s) in (\"\")"=w220) -> ("States Out"=w221:string)  [unwired: 13 in]
          }
          event Panel Close? {
            # "Discard the event because we'll close the front panel ourselves in Macro: Exit"
            # "Close Panel button (pressed) Event\n(this executes Macro: Exit to terminate the VI)"
            n123 = event-data() -> ()  [unwired: 1 in, 1 out]
            n124 = call <vilib>:"Add State(s) to Queue__jki_lib_state_machine.vi"("State(s) in Front (\"\")"="Macro: Exit", "State(s) in (\"\")"=w229) -> ("States Out"=w228:string)  [unwired: 13 in]
            n125 = event-data("Discard?"=TRUE) -> ()  [unwired: 1 in, 1 out]
          }
        }
      }
      frame "SetTogglesJet" {
        n126 = Greater?(x="Amplitude.Ch 5::8", y=2.5) -> (0:w239:bool)
        n127 = Select(t=TRUE, s=w239, f=FALSE) -> (s? t:f=w236:bool)
        n128 = Greater?(x="Width.Ch 5::8", y=0.0001) -> (0:w231:bool)
        n129 = Select(t=TRUE, s=w231, f=FALSE) -> (s? t:f=w230:bool)
        n130 = local write "Jet enable"(w230) -> ()
        n131 = local write "Jet trigger"(w236) -> ()
      }
      frame "---------- Core ----------" {
        # "Do not put any code in this frame.\n(it is a separator no-op)"
        n132 = call <vilib>:"Add State(s) to Queue__jki_lib_state_machine.vi"("State(s) in (\"\")"=w248) -> ("States Out"=w247:string)  [unwired: 14 in]
      }
      frame Default {
        w258 = 42 items=["No error", "Argument error", "Memory is full", "Out of zone", "End of file", "File already open", "Generic file I/O error", "File not found", "File permission error", "Disk is full", "Duplicate path", "Too many files open", "System feature not enabled", "Resource file not found", "Cannot add resource", "Resource not found", "Image not found", "Image memory error", "Pen does not exist", "Config type invalid", "Config token not found", "Config parse error", "Config memory error", "Bad external code format", "Bad external code offset", "External code not present", "Null window", "Destroy window error", "Null menu", "Print aborted", "Bad print record", "Print driver error", "Windows error during printing", "Memory error during printing", "Print dialog error", "Generic print error", "Invalid device refnum", "Device not found", "Device parameter error", "Device unit error", "Cannot open device", "Device call aborted", "Generic error", "Cancelled by user", "Object ID too low", "Object ID too high", "Object not in heap", "Unknown heap", "Unknown object (invalid DefProc)", "Unknown object (DefProc not in table)", "Message out of range", "Invalid (null) method", "Unknown message", "Manager call not supported", "Bad address", "Network operation in progress", "Network operation timed out", "Connection is busy", "Network attribute not supported", "Network error", "Address in use", "System out of memory", "Connection aborted", "Connection refused", "Not connected", "Already connected", "Connection closed", "Initialization error (interapplication manager)", "Bad occurrence", "Wait on unbound occurrence handler", "Occurrence queue overflow", "Datalog type conflict", "Unused", "Unrecognized type (interapplication manager)", "Memory corrupt", "Failed to make temporary DLL", "Old CIN version", "Drag socket not found", "Failed to load drop-object", "Failed to register OLE object", "Failed to release OLE object", "Format specifier type mismatch", "Unknown format specifier", "Too few format specifiers", "Too many format specifiers", "Scan failed", "Newer CIN version", "Error converting to variant", "Runtime menu error", "Password tampered", "Variant attribute not found", "Incompatible variant data type", "Event data is not available", "Event Store is not present", "Occurrence is not found", "Event Queue is not created", "Event info is not available", "Refnum passed is NULL", "Error retrieving Class GUID", "Error retrieving CoClass GUID", "Error retrieving TypeLib GUID.", "Bad built application magic bytes.", "Specific driver is different from the specific driver associated with the Logical Name.", "There is no session opened to the class driver.", "Max Error", "MAX - Error with config objects", "MAX - Error loading configuration", "MAX - Group not supported"]
        # "Current State"
        # "Do not delete, rename, or modify this frame.\n(this is used to capture unhandled states and typos)"
        # "Handle mistyped state name (developer tool)"
        n133 = Format Into String(format string="Software Exception: Unhandled State \"%s\"." ("message"), error in=w254, w249) -> (resulting string=w257:string, error out=w256:errorcluster)  [unwired: 1 in]
        n134 = call <vilib>:"Error Cluster From Error Code.vi"("show call chain? (False)"=TRUE, "error in (no error)"=w256, "error message (\"\")"=w257, "error code (0)"=w258) -> ("error out"=w255:errorcluster)  [unwired: 5 in]
        n135 = call <vilib>:"Add State(s) to Queue__jki_lib_state_machine.vi"("State(s) in (\"\")"=w253) -> ("States Out"=w252:string)  [unwired: 14 in]
      }
      frame "Initialize Core Data" {
        # "Do not delete, rename, or modify this frame.\n(this is used to determine panel behavior on exit)"
        # "originally closed?"
        # "exe?"
        # "If panel starts closed or is an EXE, then close it when we exit"
        n136 = property class="VI"() -> ("Front Panel.Open"=w267:bool)  [unwired: 2 in, 2 out]
        n137 = property class="App"() -> ("App.Kind"=w266:T4)  [unwired: 2 in, 2 out]
        n138 = control-ref of="Current VI Reference"() -> (w260:refnum<vi>)
        n139 = Not(x=w267) -> (.not. x?=w264:bool)
        n140 = Equal?(x=w266, y=T4."Run Time System" ("Application:Kind")) -> (x = y?=w263:bool)
        n141 = Or(x=w264, y=w263) -> (x .or. y?=w261:bool)
        n142 = Bundle By Name(cluster=w262, "Core.Current VI Reference"=w260, "Core.Close Panel on Exit?"=w261) -> (w269:T6)
        n143 = call <vilib>:"Add State(s) to Queue__jki_lib_state_machine.vi"("State(s) in (\"\")"=w271) -> ("States Out"=w270:string)  [unwired: 14 in]
      }
      frame "Error Handler" {
        # "Unhandled Error -- Display it"
        # "Handle any errors here.\nYou can also output any states to clean-up after errors occur"
        # "Clear error"
        n144 = call <vilib>:"General Error Handler.vi"("error in (no error)"=w273) -> ()  [unwired: 10 in, 5 out]
        n145 = call <vilib>:"Add State(s) to Queue__jki_lib_state_machine.vi"("State(s) in Front (\"\")"="/* Post Error States", "State(s) in (\"\")"=w277) -> ("States Out"=w276:string)  [unwired: 13 in]
      }
      frame "Exit" {
        # "Do not put any code in this frame.\n(No errors that occur here will be handled.)"
        n146 = call <vilib>:"Add State(s) to Queue__jki_lib_state_machine.vi"("State(s) in (\"\")"=w282) -> ("States Out"=w281:string)  [unwired: 14 in]
      }
      frame "---------- Data ----------" {
        # "Do not put any code in this frame.\n(It is a separator no-op. You can make a copy of this frame to create a new Data frame)"
        n147 = call <vilib>:"Add State(s) to Queue__jki_lib_state_machine.vi"("State(s) in (\"\")"=w286) -> ("States Out"=w285:string)  [unwired: 14 in]
      }
      frame "Data: Initialize" {
        w287 = FALSE  # Jet enable
        w288 = FALSE  # Fire Continues Allowed
        w290 = u32 0  # Tik1
        w289 = u32 0  # Tik2
        w291 = FALSE  # Jet trigger
        w292 = 0.0  # Discharge timing offset
        w293 = 0.0  # Heater timing offset
        w294 = T7 {"Current VI Reference"=refnum, "Close Panel on Exit?"=FALSE}  # Core
        # "do not delete - used by framework"
        # "Expand Bundle to add new data elements to shift register data."
        # "Add new data here."
        # "Data names and types of shift register data are defined by this bundle."
        # "Initialize the shift-register data, here.\n(data names are defined by what you wire into the bundle function)"
        n148 = Bundle("Core"=w294, "Heater timing offset"=w293, "Discharge timing offset"=w292, "Jet trigger"=w291, "Tik1"=w290, "Tik2"=w289, "Fire Continues Allowed"=w288, "Jet enable"=w287) -> (w296:T6)  [unwired: 1 in]
        n149 = call <vilib>:"Add State(s) to Queue__jki_lib_state_machine.vi"("State(s) in (\"\")"=w298) -> ("States Out"=w297:string)  [unwired: 14 in]
      }
      frame "Data: Cleanup" {
        # "Cleanup any data and references, here.\n(this is called automatically, by the Macro: Exit)"
        n150 = Unbundle By Name(w299) -> ("Core.Current VI Reference"=w302:refnum<vi>)
        n151 = Close Reference(reference=w302, error in (no error)=w301) -> (error out=w300:errorcluster)
        n152 = call <vilib>:"Add State(s) to Queue__jki_lib_state_machine.vi"("State(s) in (\"\")"=w304) -> ("States Out"=w303:string)  [unwired: 14 in]
      }
      frame "---------- UI ----------" {
        # "Do not put any code in this frame.\n(It is a separator no-op. You can make a copy of this frame to create a new UI frame)"
        n153 = call <vilib>:"Add State(s) to Queue__jki_lib_state_machine.vi"("State(s) in (\"\")"=w308) -> ("States Out"=w307:string)  [unwired: 14 in]
      }
      frame "UI: Initialize" {
        # "Initialize the User Interface, here.\n(this is called automatically, by the Macro: Init)"
        n154 = call <vilib>:"Add State(s) to Queue__jki_lib_state_machine.vi"("State(s) in (\"\")"=w312) -> ("States Out"=w311:string)  [unwired: 14 in]
      }
      frame "UI: Cursor Set" {
        # "Argument"
        # "Set and Unset Cursor Busy.\n(Usage: \"UI: Cursor Set >> Busy|Idle\")"
        n155 = case shown="\"Idle\", Default" w313 {
          tunnel: w315 -> [w320 w322]
          tunnel: [w319 w321] -> w314
          frame "Idle", Default {
            n156 = call <vilib>:"Unset Busy.vi"("error in (no error)"=w320) -> ("error out"=w319:errorcluster)  [unwired: 10 in]
          }
          frame "Busy" {
            n157 = call <vilib>:"Set Busy.vi"("error in (no error)"=w322) -> ("error out"=w321:errorcluster)  [unwired: 9 in, 1 out]
          }
        }
        n158 = call <vilib>:"Add State(s) to Queue__jki_lib_state_machine.vi"("State(s) in (\"\")"=w318) -> ("States Out"=w317:string)  [unwired: 14 in]
      }
      frame "UI: Front Panel State" {
        # "Argument"
        # "Set Front Panel Open or Closed\n(Usage: \"UI: Front Panel State >> Open|Close\")"
        n159 = Unbundle By Name(w325) -> ("Core.Current VI Reference"=w324:refnum<vi>)
        n160 = case shown="\"Close\"" w323 {
          tunnel: w327 -> [w333 w346]
          tunnel: [w335 w347] -> w326
          tunnel: w324 -> [w334 w344]
          frame "Open", Default {
            n161 = property class="VI"(reference=w334, error in=w333) -> (reference out=w331:refnum<vi>, error out=w332:errorcluster, "Front Panel.Open"=w330:bool)
            n162 = case shown="False" w330 {
              tunnel: [w338 w341] -> w335
              tunnel: w332 -> [w337 w341]
              tunnel: w331 -> [w336 _]
              frame False {
                n163 = invoke class="VI" method="FP.Open"(reference=w336, error in=w337, "Activate"=TRUE, "State"=T5."Standard") -> (error out=w338:errorcluster)  [unwired: 1 in, 4 out]
              }
              frame True {
              }
            }
          }
          frame "Close" {
            n164 = property class="VI"(reference=w344, error in=w346) -> (reference out=w343:refnum<vi>, error out=w345:errorcluster, "Front Panel.Open"=w342:bool)
            n165 = case shown="True" w342 {
              tunnel: [w348 w351] -> w347
              tunnel: w345 -> [w348 w350]
              tunnel: w343 -> [_ w349]
              frame False {
              }
              frame True {
                n166 = invoke class="VI" method="FP.Close"(reference=w349, error in=w350) -> (error out=w351:errorcluster)  [unwired: 1 in, 2 out]
              }
            }
          }
        }
        n167 = call <vilib>:"Add State(s) to Queue__jki_lib_state_machine.vi"("State(s) in (\"\")"=w329) -> ("States Out"=w328:string)  [unwired: 14 in]
      }
      frame "---------- Macro ----------" {
        # "Do not put any code in this frame.\n(It is a separator no-op. You can make a copy of this frame to create a new Macro frame)"
        n168 = call <vilib>:"Add State(s) to Queue__jki_lib_state_machine.vi"("State(s) in (\"\")"=w355) -> ("States Out"=w354:string)  [unwired: 14 in]
      }
      frame "Macro: Initialize" {
        w356 = "Data: Initialize\nInitialize Core Data\nUI: Initialize\nUI: Front Panel State >> Open"  # Data: Initialize Initialize Core Data UI: Initialize UI: Front Panel State >> Open
        # "Initialization Macro\n(This is called once, when the VI starts)"
        n169 = call <vilib>:"Add State(s) to Queue__jki_lib_state_machine.vi"("State(s) in Front (\"\")"=w356, "State(s) in (\"\")"=w360) -> ("States Out"=w359:string)  [unwired: 13 in]
      }
      frame "Macro: Exit" {
        # "Exit Macro\n(This is called once, when the VI exits)"
        n170 = Unbundle By Name(w367) -> ("Core.Close Panel on Exit?"=w366:bool)
        n171 = Select(t="UI: Front Panel State >> Close", s=w366, f="") -> (s? t:f=w363:string)
        n172 = call <vilib>:"Add State(s) to Queue__jki_lib_state_machine.vi"("State(s) in (\"\")"=w363, "State(s) at Back (\"\")"="Data: Cleanup\nExit") -> ("States Out"=w361:string)  [unwired: 13 in]
        n173 = call <vilib>:"Add State(s) to Queue__jki_lib_state_machine.vi"("State(s) in Front (\"\")"=w361, "State(s) in (\"\")"=w370) -> ("States Out"=w369:string)  [unwired: 13 in]
      }
      frame "---------- New Category ----------" {
        # "Template Separator\n(You can make a copy of, or modify, this frame)"
        n174 = call <vilib>:"Add State(s) to Queue__jki_lib_state_machine.vi"("State(s) in (\"\")"=w374) -> ("States Out"=w373:string)  [unwired: 14 in]
      }
      frame "Action: Fire" {
        # "Your code here.\n(You can make a copy of, or modify, this frame)"
        n175 = property on="fire::10" class="Str"(error in=w376, "Val(Sgnl)"="fire>>force" ("Value (Signaling)")) -> (error out=w375:errorcluster)  [unwired: 1 in, 1 out]
        n176 = call <vilib>:"Add State(s) to Queue__jki_lib_state_machine.vi"("State(s) in (\"\")"=w380) -> ("States Out"=w379:string)  [unwired: 14 in]
      }
    }
  }
